vi "Get Path Regex.vi"(8 "error in (no error)":errorcluster, 11 "InfoController in":refnum<class "InfoController.lvclass">) -> (0 "error out":errorcluster, 2 "Path Regex":string, 3 "InfoController out":refnum<class "InfoController.lvclass">)   [LabVIEW 2020, in "Vecto.lvlib" / "InfoController.lvclass"]
uses:
  InfoController.lvclass
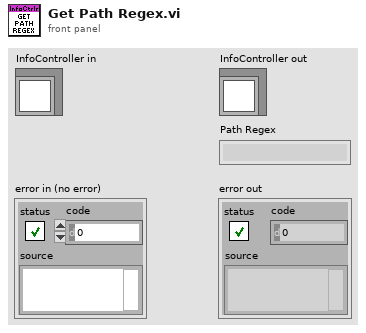
[diagram p1: front panel]
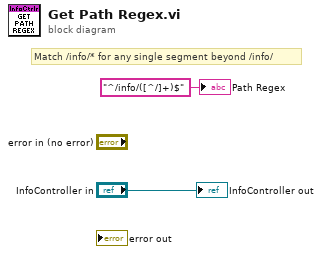
[diagram p0: block diagram]
diagram:
  # "Match /info/* for any single segment beyond /info/"
  "InfoController out" <- "InfoController in"
  "Path Regex" <- "^/info/([^/]+)$" ("Path Regex")
